vi "DriftFileHeaderV2 (SubVI).vi"(0 "Start value (V)":sgl, 1 "Byte Stream File in":refnum<file>, 3 "Settings":T1={"Drift Correction Settings"={"Drift Correction every"=80, "Drift correction Pixels"=256, "Channel index (0-23)"=0, "MaxImagesBack"=2, "Threshold"=2, "Increment"=8, "max applied Drift Correction"=20, "Correct Drift"=TRUE, "Correlate"=0, "Correct z drift"=FALSE, "zdrift \nDuration (s)"=0.0}, "Spectroscopy Setting"={"Imaging Current"=1e-11, "ref Current"=7e-11, "tip Speed (m/s)"=2e-09, "Imaging Bias"=0.02, "ref Bias"=-0.1, "preSTS delay [ms]"=500, "STS z offset"=2e-10, "during Spec Bias (V)"=-0.1, "trigger1 < Hz"=0.0, "trigger 2 >Hz"=0.0, "autoStop"=FALSE, "Spectroscopy"=0, "PLL ON/OFF"=TRUE, "readjust setpoint every "=1, "z Reference"=FALSE, "Lock In"=TRUE}, "Misc"={"File name"="symmetric_node_zOff=200p", "Email when finished"="cornelius.krull@monash.edu,Dhaneesh.Gopalakrishnan@monash.edu,marina.castelli@monash.edu"}, "Grid Settings"={"type"=1, "type order"=1, "X pixel"=0.0, "Y pixel"=0.0, "Grid_Parms"={"center X (m)"=0.0, "center Y (m)"=0.0, "width (m)"=0.0, "height (m)"=0.0, "angle (deg)"=0.0}}} {"Grid Settings"."type order" items=["Line", "Grid"]; "Grid Settings"."type" items=["Line", "Grid"]; "Spectroscopy Setting"."Spectroscopy" items=["Bias", "zSpec"]; "Spectroscopy Setting"."trigger 2 >Hz" format="%#_6p"; "Spectroscopy Setting"."trigger1 < Hz" format="%#_6p"; "Spectroscopy Setting"."during Spec Bias (V)" format="%#_5p"; "Spectroscopy Setting"."STS z offset" format="%#_6p"; "Spectroscopy Setting"."ref Bias" format="%#_6p"; "Spectroscopy Setting"."Imaging Bias" format="%#_6p"; "Spectroscopy Setting"."tip Speed (m/s)" format="%.2p"; "Spectroscopy Setting"."ref Current" format="%#_6p"; "Spectroscopy Setting"."Imaging Current" format="%#_6p"; "Drift Correction Settings"."Correlate" items=["first Frame", "successive Frames"]; "Drift Correction Settings"."max applied Drift Correction" min=1 max=100 step=1 format="%.0p"; "Drift Correction Settings"."Threshold" min=1 step=1; "Drift Correction Settings"."Channel index (0-23)" items=["Current"=0, "Z (m)"=14]}, 5 "End of Sweep":T4, 7 "Application ref in":refnum<vi>, 9 "End value (V)":sgl, 11 "error in (no error)":errorcluster, 12 "Sweep Timing":T2, 14 "Initialization":T3) -> (4 "Byte Stream File out":refnum<file>, 8 "Application ref out":refnum<vi>, 15 "error out":errorcluster)   [LabVIEW 2021]
panel:
  # "z Spectroscopy"
  # "GRID points"
  # "Increase this if no Drift was detected for \na certain number of images"
  # "% of image size"
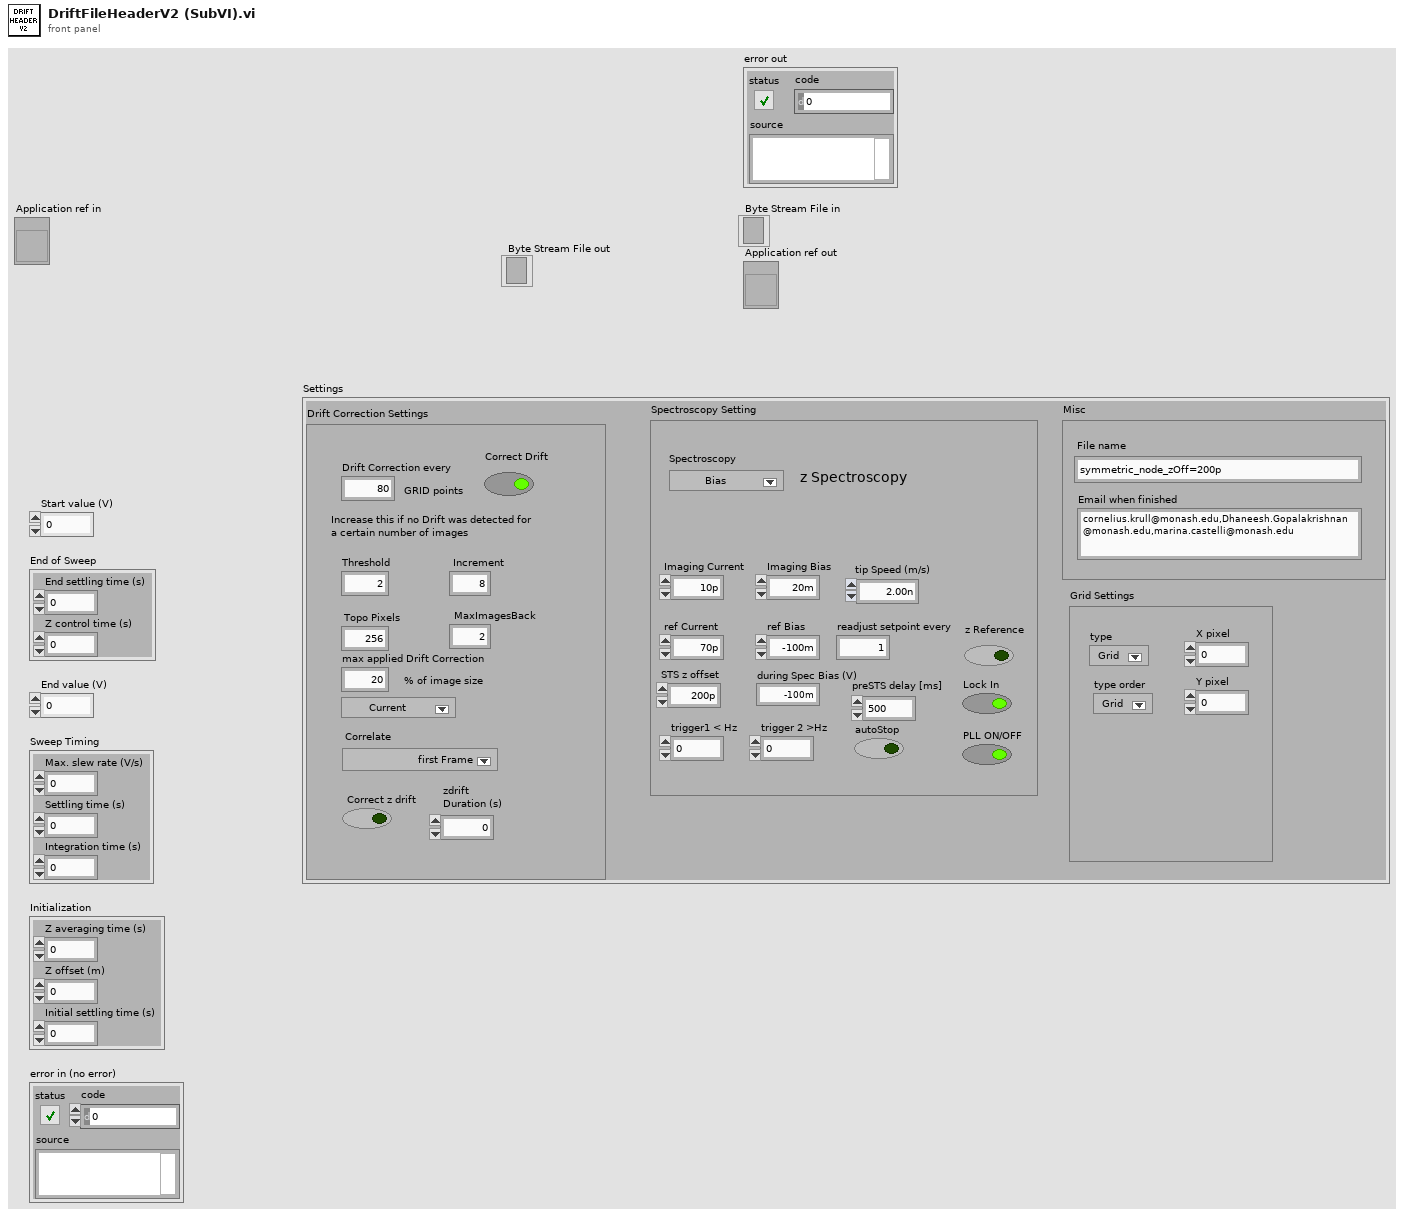
[diagram p1: front panel]
types:
  T1 = cluster{"Drift Correction Settings":cluster{"Drift Correction every":i32, "Drift correction Pixels":i32, "Channel index (0-23)":u8, "MaxImagesBack":i32, "Threshold":i32, "Increment":i32, "max applied Drift Correction":i32, "Correct Drift":bool, "Correlate":u16, "Correct z drift":bool, "zdrift \nDuration (s)":dbl}, "Spectroscopy Setting":cluster{"Imaging Current":dbl, "ref Current":dbl, "tip Speed (m/s)":sgl, "Imaging Bias":dbl, "ref Bias":dbl, "preSTS delay [ms]":u32, "STS z offset":dbl, "during Spec Bias (V)":sgl, "trigger1 < Hz":sgl, "trigger 2 >Hz":sgl, "autoStop":bool, "Spectroscopy":u16, "PLL ON/OFF":bool, "readjust setpoint every ":i32, "z Reference":bool, "Lock In":bool}, "Misc":cluster{"File name":string, "Email when finished":string}, "Grid Settings":cluster{"type":u16, "type order":u16, "X pixel":dbl, "Y pixel":dbl, "Grid_Parms":cluster{"center X (m)":sgl, "center Y (m)":sgl, "width (m)":sgl, "height (m)":sgl, "angle (deg)":sgl}}}
  T2 = cluster{"Max. slew rate (V/s)":sgl, "Settling time (s)":sgl, "Integration time (s)":sgl}
  T3 = cluster{"Z averaging time (s)":sgl, "Z offset (m)":sgl, "Initial settling time (s)":sgl}
  T4 = cluster{"End settling time (s)":sgl, "Z control time (s)":sgl}
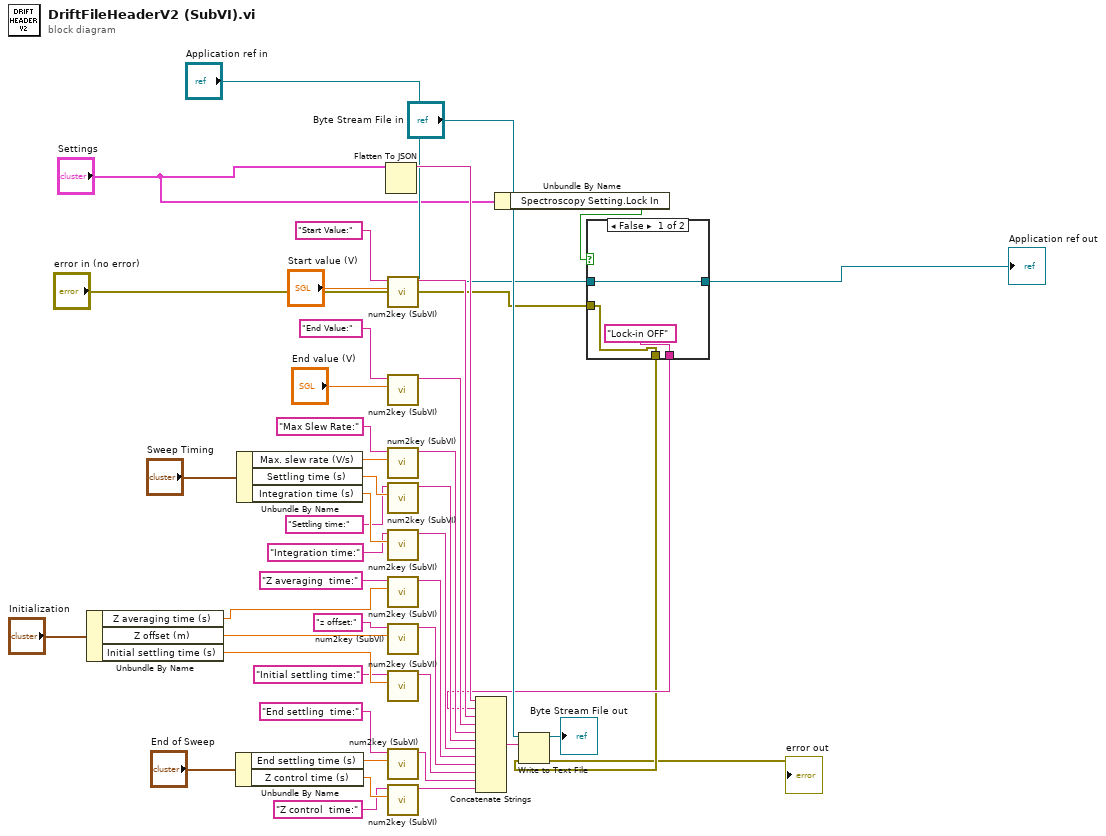
[diagram p0: block diagram]
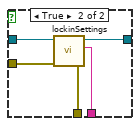
[diagram p2: hidden frame]
diagram:
  n1 = Unbundle By Name("Initialization") -> ("Z averaging time (s)"=w28:sgl, "Z offset (m)"=w27:sgl, "Initial settling time (s)"=w30:sgl)
  n2 = Unbundle By Name("End of Sweep") -> ("End settling time (s)"=w34:sgl, "Z control time (s)"=w33:sgl)
  n3 = Unbundle By Name("Sweep Timing") -> ("Max. slew rate (V/s)"=w20:sgl, "Settling time (s)"=w21:sgl, "Integration time (s)"=w22:sgl)
  n4 = Flatten To JSON(anything="Settings") -> (JSON string=w9:string)  [unwired: 2 in, 1 out]
  n5 = call "num2key (SubVI).vi"("Img current"="Start value (V)", "String in"="Start Value:") -> ("String out"=w35:string)  [unwired: 9 in]
  n6 = call "num2key (SubVI).vi"("Img current"="End value (V)", "String in"="End Value:") -> ("String out"=w36:string)  [unwired: 9 in]
  n7 = call "num2key (SubVI).vi"("Img current"=w20, "String in"="Max Slew Rate:") -> ("String out"=w37:string)  [unwired: 9 in]
  n8 = call "num2key (SubVI).vi"("Img current"=w21, "String in"="Settling time:") -> ("String out"=w38:string)  [unwired: 9 in]
  n9 = call "num2key (SubVI).vi"("Img current"=w22, "String in"="Integration time:") -> ("String out"=w39:string)  [unwired: 9 in]
  n10 = call "num2key (SubVI).vi"("Img current"=w28, "String in"="Z averaging  time:") -> ("String out"=w40:string)  [unwired: 9 in]
  n11 = call "num2key (SubVI).vi"("Img current"=w27, "String in"="z offset:") -> ("String out"=w41:string)  [unwired: 9 in]
  n12 = call "num2key (SubVI).vi"("Img current"=w30, "String in"="Initial settling time:") -> ("String out"=w42:string)  [unwired: 9 in]
  n13 = call "num2key (SubVI).vi"("Img current"=w34, "String in"="End settling  time:") -> ("String out"=w43:string)  [unwired: 9 in]
  n14 = call "num2key (SubVI).vi"("Img current"=w33, "String in"="Z control  time:") -> ("String out"=w44:string)  [unwired: 9 in]
  n15 = Unbundle By Name("Settings") -> ("Spectroscopy Setting.Lock In"=w5:bool)
  n16 = case shown="False" w5 {
    tunnel: "Application ref in" -> [w48 w53]
    tunnel: [w48 w52] -> w7
    tunnel: ["Lock-in OFF" ("concatenated string") w51] -> w4
    tunnel: "error in (no error)" -> [w46 w50]
    tunnel: [w46 w49] -> w2
    frame False {
    }
    frame True {
      n17 = call "lockinSettings.vi"("Error in (no error)"=w50, "Application ref in"=w53) -> ("Error out"=w49:errorcluster, "concatenated string"=w51:string, "Application ref out"=w52:refnum<vi>)  [unwired: 5 in]
    }
  }
  "Application ref out" <- w7
  n18 = Concatenate Strings(w9, w4, w35, w36, w37, w38, w39, w40, w41, w42, w43, w44) -> (w45:string)
  n19 = Write to Text File(file (use dialog)="Byte Stream File in", text=w45, error in=w2) -> (refnum out=→"Byte Stream File out":refnum<file>, error out=→"error out":errorcluster)  [unwired: 1 in, 1 out]
